vi "Test - Child Class Serialization.vi"(8 "error in":errorcluster) -> (0 "error out":errorcluster)   [LabVIEW 2020, in "TEST - JKI JSON Object Serialization.lvlib"]
uses:
  TEST - JKI JSON Object Serialization.lvlib
  support/Child/Child.lvclass
  C:/projects/JKI-JSON-Object-Serialization/tests/support/Parent/Parent.lvclass
  support/Child/Child.lvclass/Child.ctl
  support/Parent/Parent.lvclass/Parent.ctl
  <vilib>/addons/_JKI Toolkits/Caraya/classes/Test/Test.lvclass
  source/library/JKI JSON Object Serialization.lvlib
  support/Parent/Parent.lvclass
  <vilib>/addons/_JKI Toolkits/Caraya/classes/Assert/Assert.lvclass
panel:
  out "JSON String":string
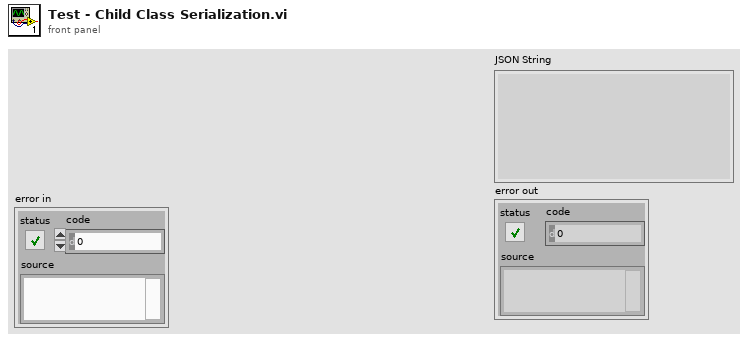
[diagram p1: front panel]
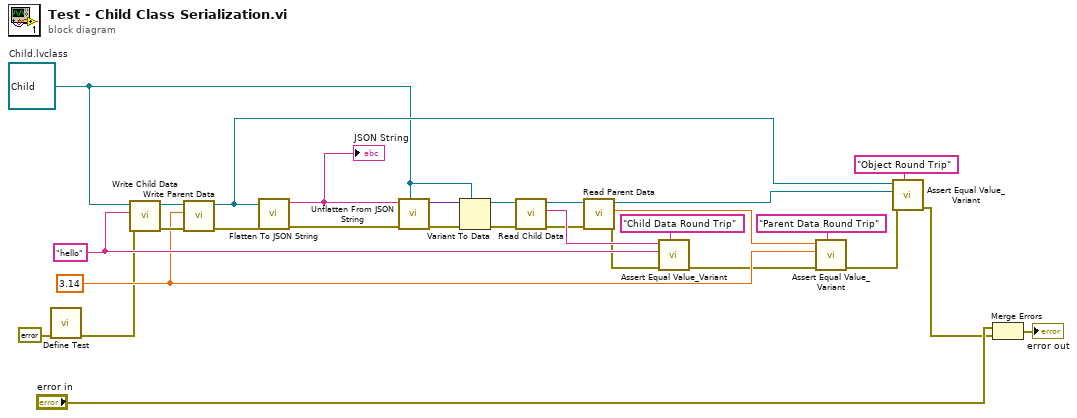
[diagram p0: block diagram]
diagram:
  w13 = 3.14 ("Parent Data")
  w16 = "hello" ("Child Data")
  w1 = refnum<class "Child.lvclass"> refnum  # Child.lvclass
  n1 = call <vilib>:"Define Test.vi"("error in (no error)"=errorcluster {"status"=FALSE, "code"=0, "source"=""}) -> ("error out"=w9:errorcluster)  [unwired: 9 in, 1 out]
  n2 = call "Write Child Data.vi"("error in (no error)"=w9, "Child Data"=w16, "Child in"=w1) -> ("error out"=w25:errorcluster, "Child out"=w26:refnum<class "Child.lvclass">)  [unwired: 7 in]
  n3 = call "Write Parent Data.vi"("error in (no error)"=w25, "Parent Data"=w13, "Parent in"=w26) -> ("error out"=w24:errorcluster, "Parent out"=w2:refnum<class "Child.lvclass">)  [unwired: 7 in]
  n4 = call "Flatten To JSON String.vi"("error in (no error)"=w24, "Variant"=w2) -> ("error out"=w22:errorcluster, "JSON String"=w23:string)  [unwired: 8 in]
  "JSON String" <- w23
  n5 = call "Unflatten From JSON String.vi"("Type and Defaults"=w1, "error in (no error)"=w22, "JSON String"=w23) -> ("error out"=w21:errorcluster, "Variant"=w20:variant)  [unwired: 7 in]
  n6 = Variant To Data(error in=w21, type=w1, Variant=w20) -> (data=w19:refnum<class "Child.lvclass">, error out=w15:errorcluster)
  n7 = call "Read Child Data.vi"("error in (no error)"=w15, "Child in"=w19) -> ("error out"=w12:errorcluster, "Child Data"=w17:string, "Child out"=w18:refnum<class "Child.lvclass">)  [unwired: 7 in]
  n8 = call "Read Parent Data.vi"("error in (no error)"=w12, "Parent in"=w18) -> ("error out"=w11:errorcluster, "Parent Data"=w14:dbl, "Parent out"=w6:refnum<class "Child.lvclass">)  [unwired: 7 in]
  n9 = call <vilib>:"Assert Equal Value_Variant.vi"("Label"="Child Data Round Trip", "error in (no error)"=w11, "Y"=w16, "X"=w17) -> ("error out"=w10:errorcluster)  [unwired: 6 in, 1 out]
  n10 = call <vilib>:"Assert Equal Value_Variant.vi"("Label"="Parent Data Round Trip", "error in (no error)"=w10, "Y"=w13, "X"=w14) -> ("error out"=w8:errorcluster)  [unwired: 6 in, 1 out]
  n11 = call <vilib>:"Assert Equal Value_Variant.vi"("Label"="Object Round Trip", "error in (no error)"=w8, "Y"=w6, "X"=w2) -> ("error out"=w7:errorcluster)  [unwired: 6 in, 1 out]
  n12 = Merge Errors("error in", w7) -> (→"error out":errorcluster)
